vi "Clear Log Control.vi"(8 "エラー入力 (エラーなし)":errorcluster, 11 "Result Log Reference":refnum<vi>) -> (0 "エラー出力":errorcluster, 3 "Result Log Reference Out":refnum<vi>)   [LabVIEW 2020]
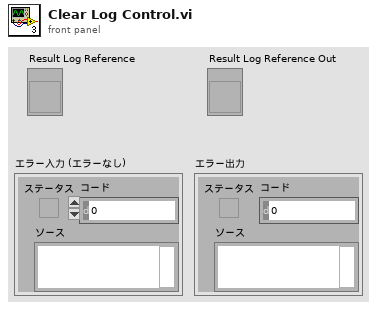
[diagram p1: front panel]
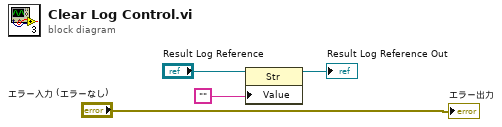
[diagram p0: block diagram]
diagram:
  n1 = property class="Str"(reference="Result Log Reference", "Value"="") -> (reference out=→"Result Log Reference Out":refnum<vi>)  [unwired: 1 in, 1 out]
  "エラー出力" <- "エラー入力 (エラーなし)"
